vi "Get Difference In Time.vi"(11 "Calculate Time Difference":bool) -> (2 "Delta Time over Time":u32(graph), 3 "Delta Time (ms)":dbl)   [LabVIEW 2018]
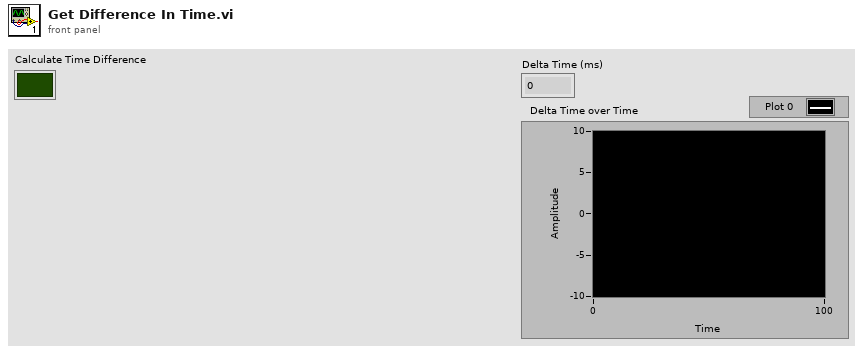
[diagram p1: front panel]
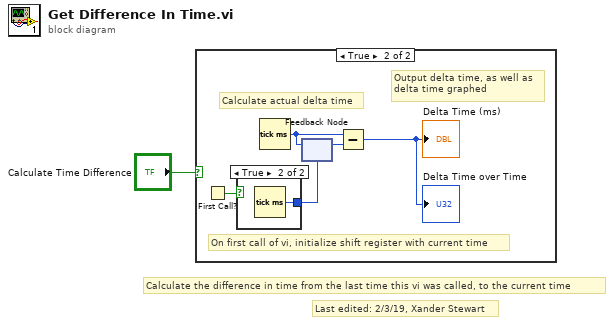
[diagram p0: block diagram]
diagram:
  # "Last edited: 2/3/19, Xander Stewart"
  # "Calculate the difference in time from the last time this vi was called, to the current time"
  n1 = case shown="True" "Calculate Time Difference" {
    frame False {
    }
    frame True {
      # "Output delta time, as well as\ndelta time graphed"
      # "Calculate actual delta time"
      # "On first call of vi, initialize shift register with current time"
      n2 = First Call?() -> (First Call?: T/F=w4:bool)
      n3 = case shown="True" w4 {
        tunnel: [_ w7] -> w3
        frame False {
        }
        frame True {
          n4 = Tick Count (ms)() -> (millisecond timer value=w7:u32)
        }
      }
      n5 = Tick Count (ms)() -> (millisecond timer value=w6:u32)
      n6 = feedback #1(w3) -> (w5:u32)
      n7 = feedback-in #1(w6) -> ()
      n8 = Subtract(x=w6, y=w5) -> (x-y=→"Delta Time (ms)" →"Delta Time over Time":u32)
    }
  }
